vi "exporting data test.vi"() -> ()   [LabVIEW 2021]
panel:
  out "Numeric 2":dbl
  out "Numeric":dbl
  in  "Therm 2 order":i32=3
  in  "Therm 2 low cutoff freq":dbl=5.0 format="%#_13g"
  in  "Therm 2 sampling freq":dbl=200.0 format="%#_13g"
  out "Thermistor 2":T1
  in  "Thermistor 2":T1
  out "Thermistor 1":T1
  in  "Thermistor 1":T1
  out "Thermistor 1 and 2":cluster{"Filtered x":dbl, "Filtered x":dbl}(graph)
  in  "Therm 1 sampling freq: fs":dbl=200.0 format="%#_13g"
  in  "Therm 1 order order":i32=3
  in  "Therm 1 low cutoff freq":dbl=5.0 format="%#_13g"
  in  "stop":bool
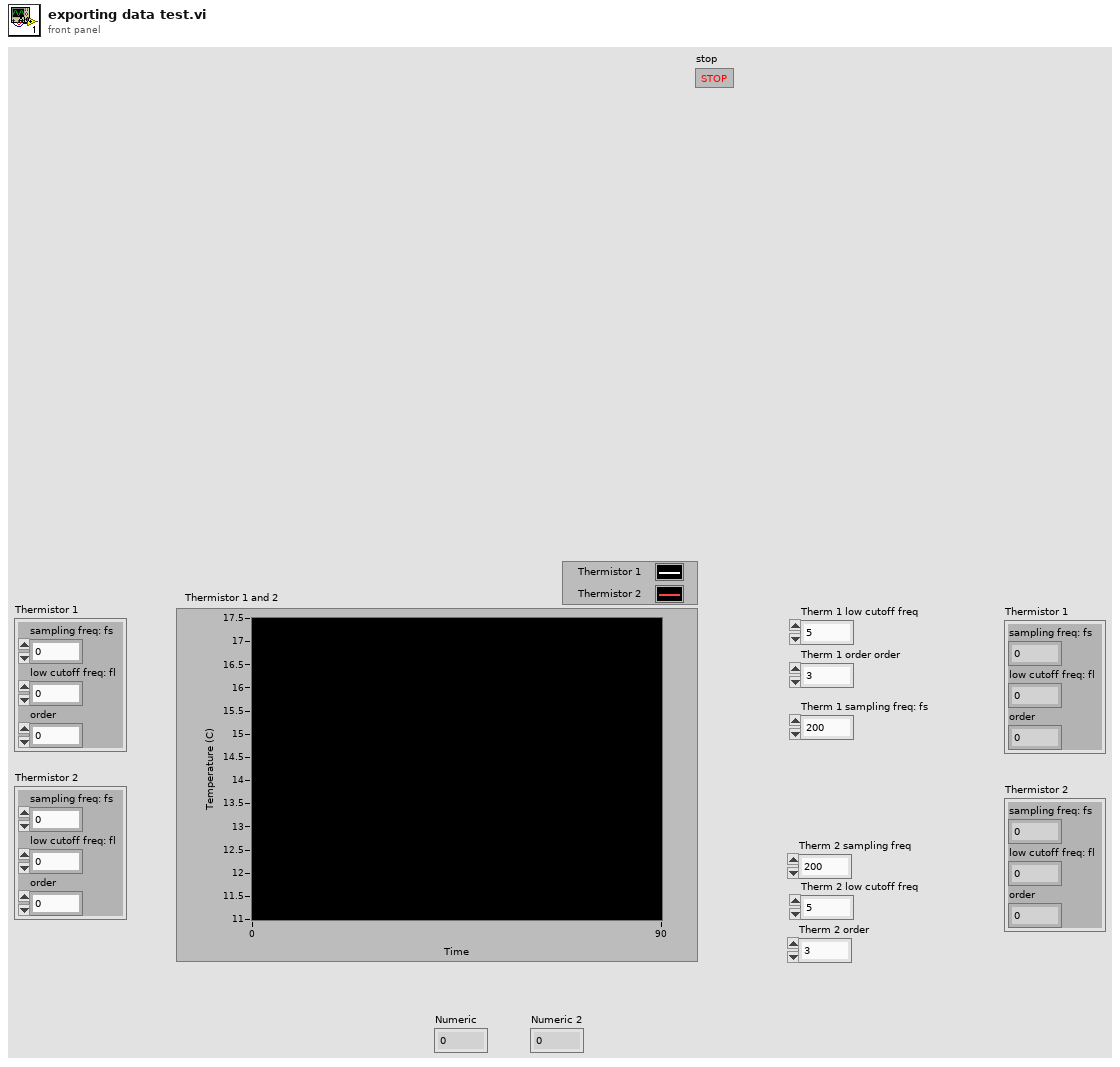
[diagram p1: front panel]
types:
  T1 = cluster{"sampling freq: fs":dbl, "low cutoff freq: fl":dbl, "order":i32}
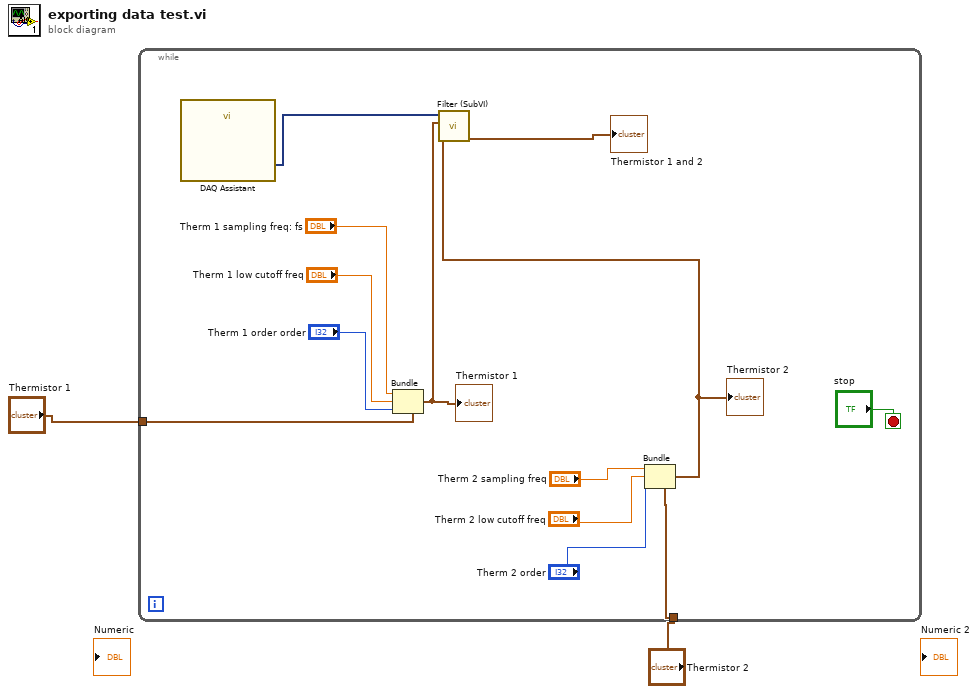
[diagram p0: block diagram]
diagram:
  n1 = while {
    tunnel: "Thermistor 1" -> [w9]
    tunnel: "Thermistor 2" -> [w7]
    stop <- "stop" stop-if-true
    n2 = call "DAQ Assistant"() -> ("data"=w14:dynamicdata)  [unwired: 17 in, 2 out]
    n3 = Bundle(cluster=w9, "sampling freq: fs"="Therm 1 sampling freq: fs", "low cutoff freq: fl"="Therm 1 low cutoff freq", "order"="Therm 1 order order") -> (w8:T1)
    "Thermistor 1" <- w8
    n4 = Bundle(cluster=w7, "sampling freq: fs"="Therm 2 sampling freq", "low cutoff freq: fl"="Therm 2 low cutoff freq", "order"="Therm 2 order") -> (w6:T1)
    "Thermistor 2" <- w6
    n5 = call "Filter (SubVI).vi"("Thermistor 2"=w6, "Thermistor 1"=w8, "data"=w14) -> ("Thermistor 1 and 2"=→"Thermistor 1 and 2":cluster{"Filtered x":dbl, "Filtered x":dbl})  [unwired: 8 in]
  }
